vi "Internal Error Class.vi"(8 "error in (no error)":errorcluster, 11 "Error Interface in":refnum<class "Error Interface.lvclass">) -> (0 "error out":errorcluster, 3 "Error Interface out":refnum<class "Error Interface.lvclass">)   [LabVIEW 2016, in "Stream Error.lvlib" / "Error Interface.lvclass"]
doc: "--\nCopyright © 2017 Composed SystemsI All rights reserved.\n\nAuthor: Jon McBee <jon.mcbee@composed.io>\n\nThis library is provided \"AS IS\" ,WITHOUT WARRANTIES OR\nCONDITIONS OF ANY KIND, either express or implied.\n\nComposed Systems -- composed.io\n\nStream 0.0.1.1\nJon McBee - Composed Systems\nCopyright (c) 2017, Composed Systems"
uses:
  <userlib>/Composed Systems/Stream/Error/Classes/Error Interface/Error Interface.lvclass
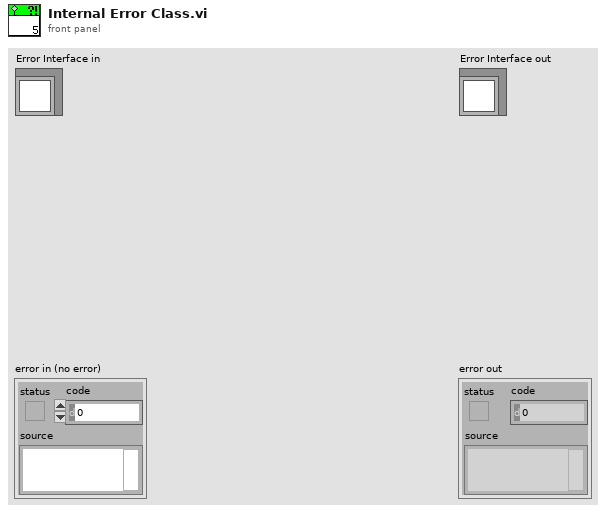
[diagram p1: front panel]
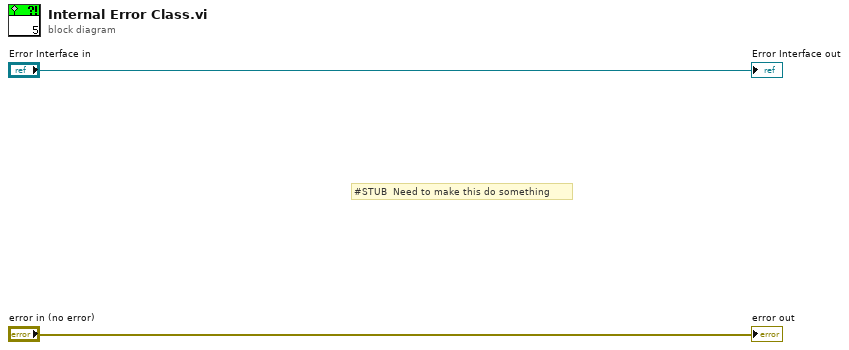
[diagram p0: block diagram]
diagram:
  # "#STUB  Need to make this do something"
  "error out" <- "error in (no error)"
  "Error Interface out" <- "Error Interface in"
